vi "ImagenSegmentada.vi"(11 "ImagenCapturadaIMAQ":T1 caption="ImagenCapturada") -> (1 "colorSegmentado":u32[][](array[numeric]), 3 "bnSegmentado":bool[][](array[boolean]))   [LabVIEW 2021]
uses:
  <vilib>/vision/Image Controls.llb/IMAQ Image.ctl
  <vilib>/picture/picture.llb/Draw 1-Bit Pixmap.vi
  <vilib>/picture/picture.llb/Draw True-Color Pixmap.vi
panel:
  out "binaria":picture
  out "color":picture caption="Color"
  in  "umbralRojo":u8
  in  "umbralVerde":u8
  in  "umbralAzul":u8
  in  "toleranciaRoja":u8=10
  in  "toleranciaAzul":u8=10
  in  "toleranciaVerde":u8=10
  # "G"
  # "B"
  # "R"
  # "UMBRAL"
  # "TOLERANCIA"
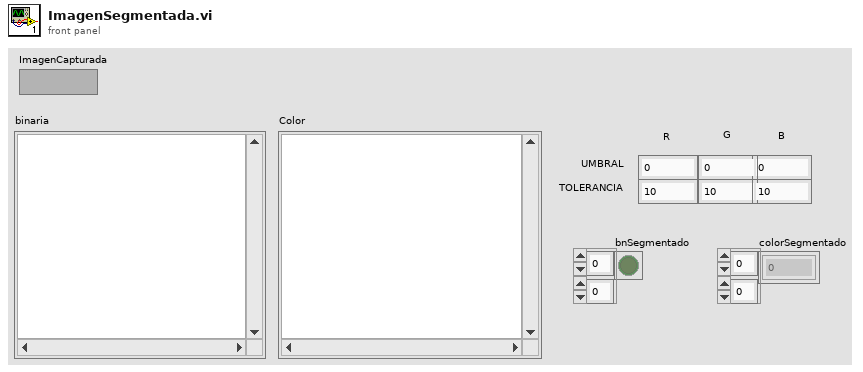
[diagram p1: front panel]
types:
  T1 = typedef "IMAQ Image.ctl" = refnum<image>
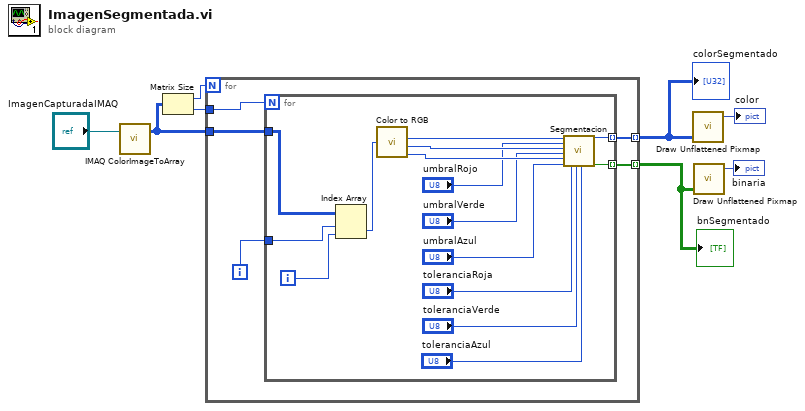
[diagram p0: block diagram]
diagram:
  n1 = call "IMAQ ColorImageToArray"("Image"="ImagenCapturadaIMAQ") -> ("Image Pixels (U32)"=w8:u32[][])  [unwired: 3 in, 2 out]
  n2 = Matrix Size(0:w8) -> (1:w7:i32, 2:w6:i32)
  n3 = for {
    N: w7 -> [_]
    tunnel: w8 -> [w13]
    tunnel: w6 -> [w12]
    tunnel: [w10] -> w3 mode=indexing
    tunnel: [w9] -> w2 mode=indexing
    i -> [w11]
    n4 = for {
      N: w12 -> [_]
      tunnel: w13 -> [w28]
      tunnel: w11 -> [w27]
      tunnel: [w15] -> w10 mode=indexing
      tunnel: [w14] -> w9 mode=indexing
      i -> [w26]
      n5 = Index Array(array=w28, index (row)=w27, index (col)=w26) -> (element=w25:u32)
      n6 = call <vilib>:"Color to RGB.vi"("Color"=w25) -> ("R"=w24:u8, "G"=w23:u8, "B"=w22:u8)  [unwired: 1 out]
      n7 = call "Segmentacion.vi"("R"=w24, "UR"="umbralRojo", "G"=w23, "UG"="umbralVerde", "B"=w22, "UB"="umbralAzul", "TR"="toleranciaRoja", "TG"="toleranciaVerde", "TB"="toleranciaAzul") -> ("ColorSegmentado"=w15:u32, "binario"=w14:bool)  [unwired: 9 in]
    }
  }
  "bnSegmentado" <- w2
  "colorSegmentado" <- w3
  n8 = call-poly <vilib>:"Draw Unflattened Pixmap.vi"("data (RGB format)"=w3) -> ("new picture"=→"color":picture)  [unwired: 8 in]
  n9 = call-poly <vilib>:"Draw Unflattened Pixmap.vi"("data"=w2) -> ("new picture"=→"binaria":picture)  [unwired: 8 in]
